vi "Fancy Swerve.vi"   [LabVIEW 2020]
uses:
  Robot Global Data.vi
  <vilib>/addons/control/pid/pid.llb/PID (DBL).vi
  <vilib>/addons/control/pid/NI_PID_pid.lvlib
types:
  T1 = cluster{"proportional gain (Kc)":dbl, "integral time (Ti, min)":dbl, "derivative time (Td, min)":dbl}
  T2 = typedef "WPI_MotorControlDeviceRef.ctl" = cluster{"DeviceStatus":errorcluster, "Type":T3, "PWM":cluster{"PWM Channel":T4, "DeadBand":T5}, "CAN":cluster{"Device Number":u8, "SetOutput VI Ref":variant, "GetOutput VI Ref":variant, "Enable VI Ref":variant, "Disable VI Ref":variant, "Data":variant}, "Invert":bool, "DIO PWM":cluster{"PWM \"Enable\" Channel":T4, "DIOChannel":T6, "PWM Rate":dbl}}
  T3 = typedef "WPI_MotorControlType.ctl" = enum16{"PWM", "CAN", "DIO PWM"}
  T4 = typedef "FPGA_DIOPWMChannel.ctl" = enum8{"PWM 0", "PWM 1", "PWM 2", "PWM 3", "PWM 4", "PWM 5", "PWM 6", "PWM 7", "PWM 8", "PWM 9", "PWM MXP 0", "PWM MXP 1", "PWM MXP 2", "PWM MXP 3", "PWM MXP 4", "PWM MXP 5", "PWM MXP 6", "PWM MXP 7", "PWM MXP 8", "PWM MXP 9", "Invalid"}
  T5 = typedef "WPI_PWMDeadband.ctl" = cluster{"Name":string, "maxPositivePwm":i32, "minPositivePwm":i32, "centerPwm":i32, "maxNegativePwm":i32, "minNegativePwm":i32, "angularRange":u16}
  T6 = typedef "FPGA_DIOChannel.ctl" = enum8{"DIO 0", "DIO 1", "DIO 2", "DIO 3", "DIO 4", "DIO 5", "DIO 6", "DIO 7", "DIO 8", "DIO 9", "DIO MXP 0", "DIO MXP 1", "DIO MXP 2", "DIO MXP 3", "DIO MXP 4", "DIO MXP 5", "DIO MXP 6", "DIO MXP 7", "DIO MXP 8", "DIO MXP 9", "DIO MXP 10", "DIO MXP 11", "DIO MXP 12", "DIO MXP 13", "DIO MXP 14", "DIO MXP 15", "SPI Port CS1", "SPI Port CS2", "SPI Port CS3", "SPI Port MISO", "SPI Port MOSI", "Invalid"}
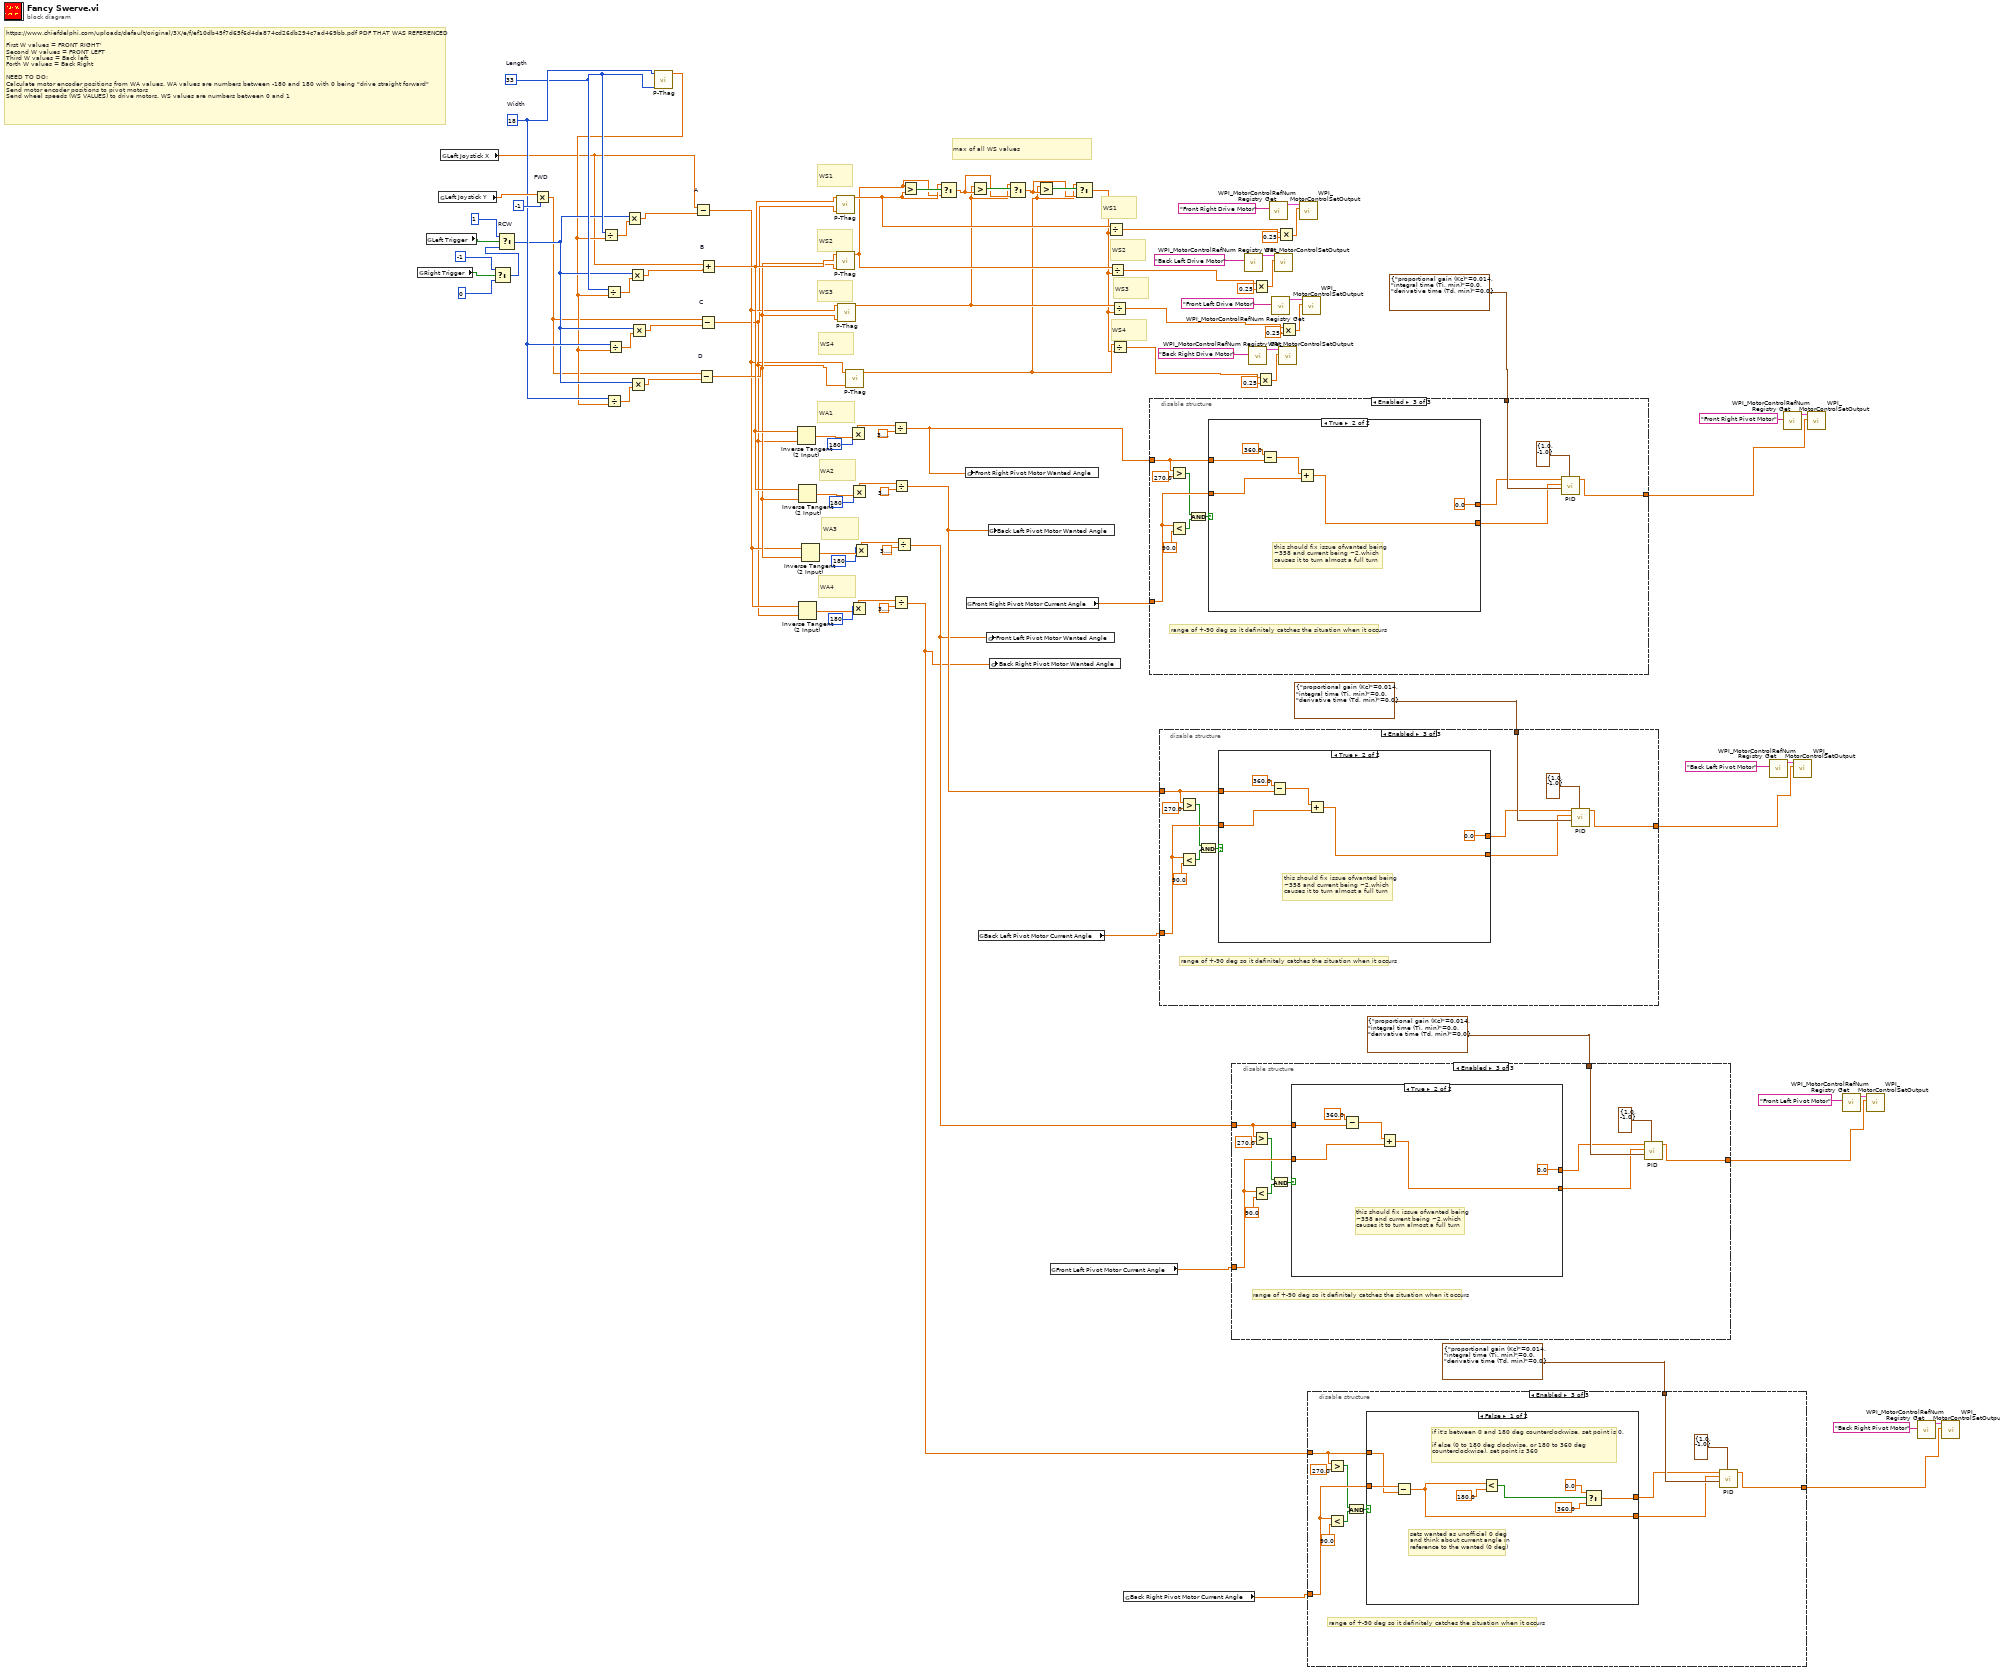
[diagram p0: block diagram]
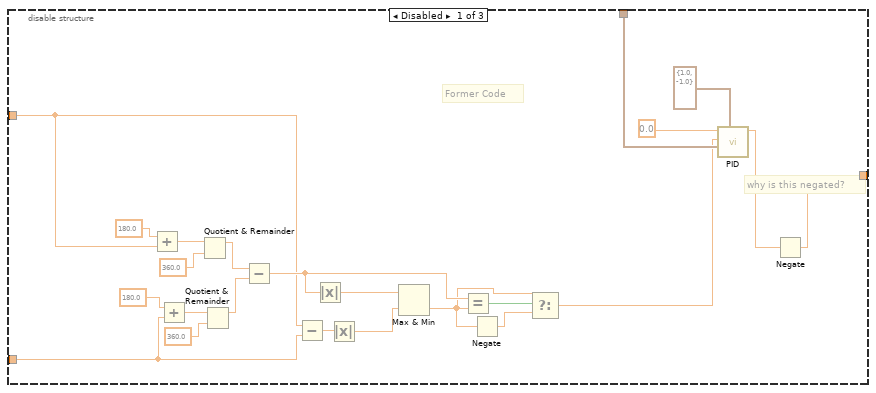
[diagram p2: hidden frame]
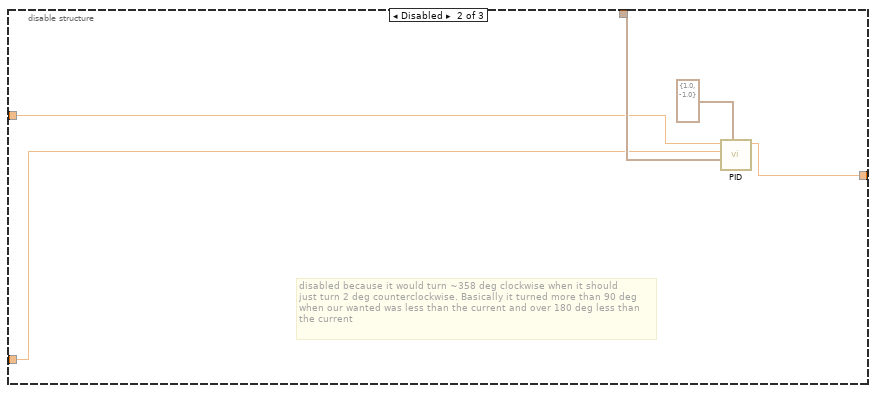
[diagram p3: hidden frame]
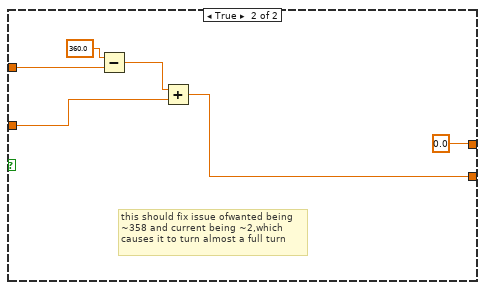
[diagram p4: hidden frame]
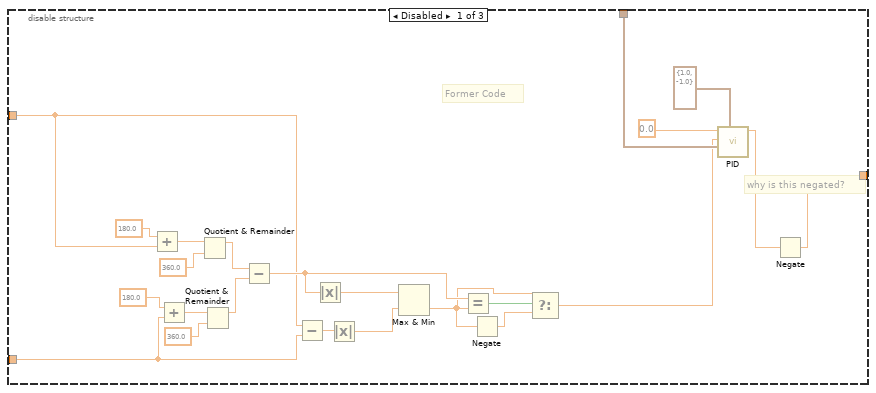
[diagram p5: hidden frame]
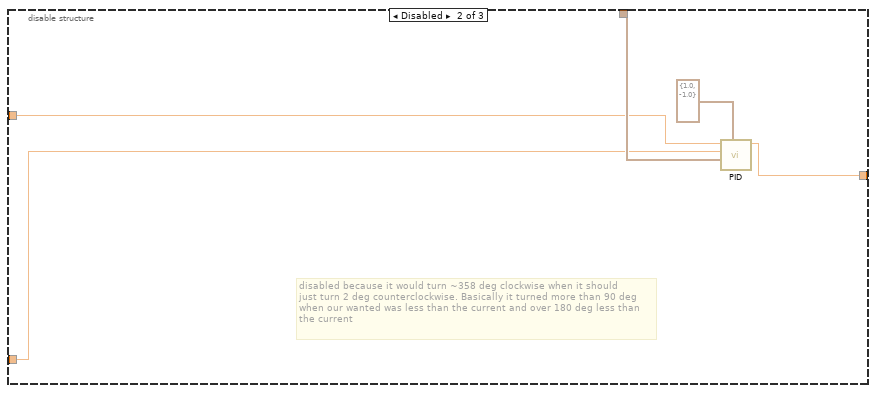
[diagram p6: hidden frame]
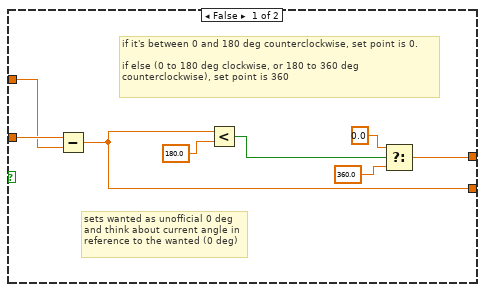
[diagram p7: hidden frame]
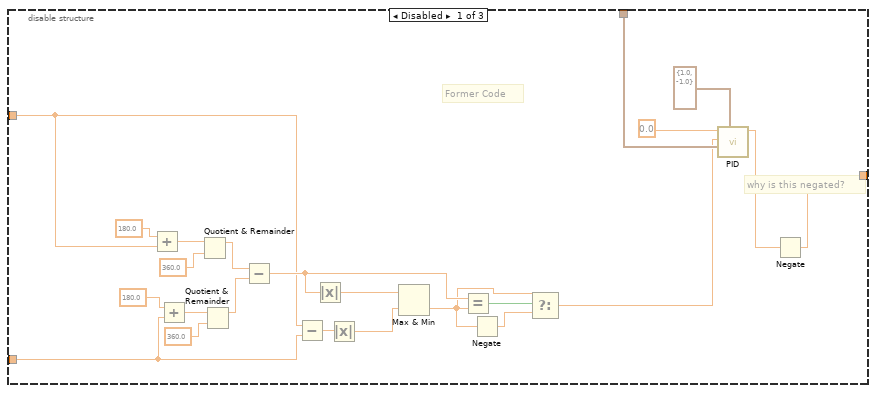
[diagram p8: hidden frame]
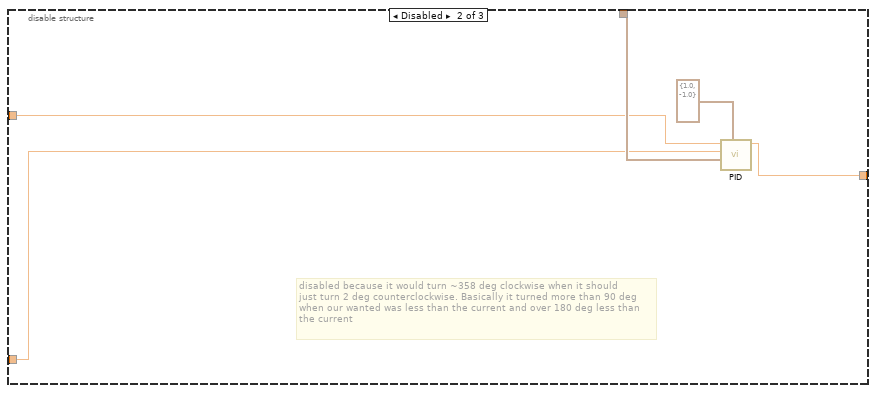
[diagram p9: hidden frame]
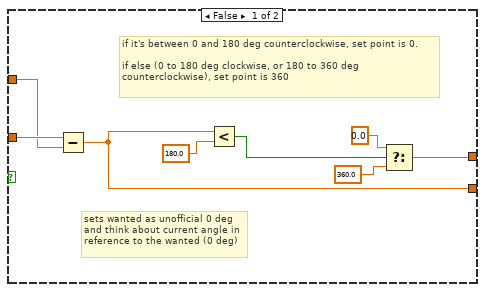
[diagram p10: hidden frame]
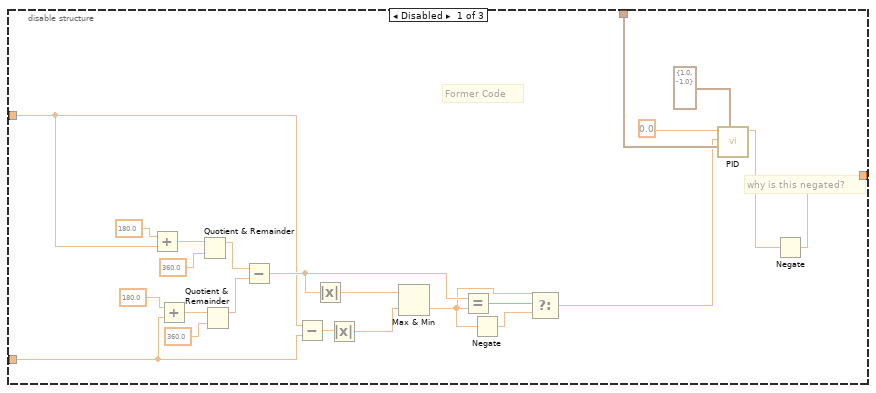
[diagram p11: hidden frame]
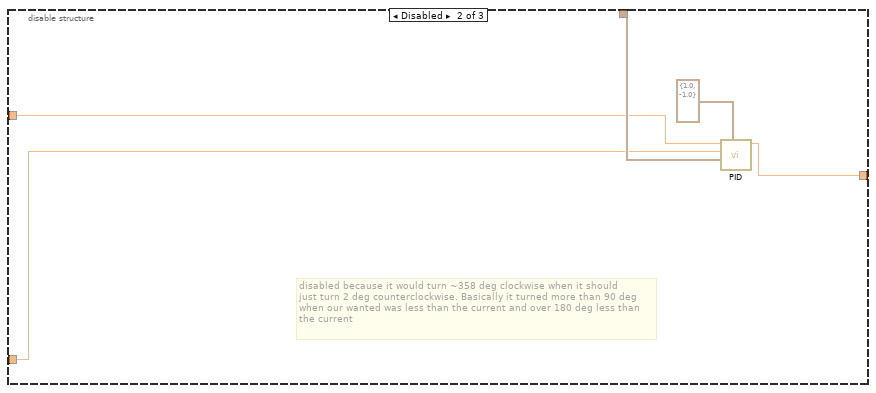
[diagram p12: hidden frame]
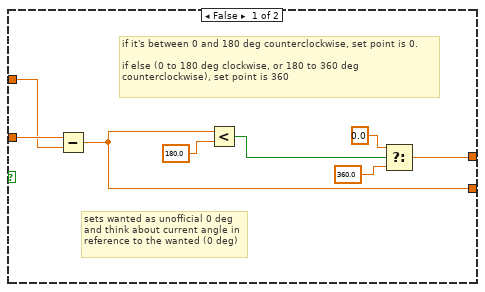
[diagram p13: hidden frame]
diagram:
  w79 = 33  # Length
  w80 = 18  # Width
  # "WS4"
  # "WS3"
  # "WS2"
  # "WS1"
  # "https://www.chiefdelphi.com/uploads/default/original/3X/e/f/ef10db45f7d65f6d4da874cd26db294c7ad469bb.pdf PDF THAT WAS REFERENCED\n\nFirst W values = FRONT RIGHT'\nSecond W values = FRONT LEFT\nThird W values = Back left\nForth W values = Back Right\n\nNEED TO DO:\nCalculate motor encoder positions from WA values. WA values are numbers between -180 and 180 with 0 being \"drive straight forward\"\nSend motor encoder positions to pivot motors\nSend wheel speeds (WS VALUES) to drive motors. WS values are numbers between 0 and 1"
  # "max of all WS values"
  # "WA4"
  # "WA3"
  # "WA2"
  # "WA1"
  # "WS4"
  # "WS3"
  # "WS2"
  # "WS1"
  n1 = global read "Robot Global Data.vi" "Right Trigger"() -> (w91:bool)
  n2 = global read "Robot Global Data.vi" "Left Trigger"() -> (w93:bool)
  n3 = global read "Robot Global Data.vi" "Left Joystick Y"() -> (w96:dbl)
  n4 = global read "Robot Global Data.vi" "Left Joystick X"() -> (w2:dbl)
  n5 = Select(t=-1, s=w91, f=0) -> (s? t:f=w92:i32)
  n6 = Select "RCW"(t=1, s=w93, f=w92) -> (s? t:f=w4:i32)
  n7 = Multiply "FWD"(x=w96, y=-1) -> (x*y=w1:dbl)
  n8 = call "P-Thag.vi"("Width"=w80, "Length"=w79) -> ("Output"=w3:dbl)  [unwired: 7 in]
  n9 = Divide(x=w79, y=w3) -> (x/y=w88:dbl)
  n10 = Divide(x=w79, y=w3) -> (x/y=w86:dbl)
  n11 = Divide(x=w80, y=w3) -> (x/y=w82:dbl)
  n12 = Divide(x=w80, y=w3) -> (x/y=w84:dbl)
  n13 = Multiply(x=w4, y=w88) -> (x*y=w87:dbl)
  n14 = Multiply(x=w4, y=w86) -> (x*y=w85:dbl)
  n15 = Multiply(x=w4, y=w82) -> (x*y=w81:dbl)
  n16 = Multiply(x=w4, y=w84) -> (x*y=w83:dbl)
  n17 = Subtract "A"(x=w2, y=w87) -> (x-y=w60:dbl)
  n18 = Subtract "D"(x=w1, y=w81) -> (x-y=w61:dbl)
  n19 = Subtract "C"(x=w1, y=w83) -> (x-y=w59:dbl)
  n20 = Add "B"(x=w2, y=w85) -> (x+y=w62:dbl)
  n21 = Inverse Tangent (2 Input)(1:w59, 2:w62) -> (0:w77:dbl)
  n22 = Inverse Tangent (2 Input)(1:w59, 2:w60) -> (0:w64:dbl)
  n23 = Inverse Tangent (2 Input)(1:w61, 2:w62) -> (0:w72:dbl)
  n24 = Inverse Tangent (2 Input)(1:w61, 2:w60) -> (0:w69:dbl)
  n25 = call "P-Thag.vi"("Width"=w62, "Length"=w59) -> ("Output"=w53:dbl)  [unwired: 7 in]
  n26 = call "P-Thag.vi"("Width"=w62, "Length"=w61) -> ("Output"=w52:dbl)  [unwired: 7 in]
  n27 = call "P-Thag.vi"("Width"=w60, "Length"=w61) -> ("Output"=w51:dbl)  [unwired: 7 in]
  n28 = call "P-Thag.vi"("Width"=w60, "Length"=w59) -> ("Output"=w50:dbl)  [unwired: 7 in]
  n29 = Multiply(x=180, y=w77) -> (x*y=w76:dbl)
  n30 = Multiply(x=180, y=w64) -> (x*y=w65:dbl)
  n31 = Multiply(x=180, y=w72) -> (x*y=w73:dbl)
  n32 = Multiply(x=180, y=w69) -> (x*y=w68:dbl)
  n33 = Divide(x=w76, y=3.141592653589793) -> (x/y=w28:dbl)
  n34 = Divide(x=w65, y=3.141592653589793) -> (x/y=w5:dbl)
  n35 = Divide(x=w73, y=3.141592653589793) -> (x/y=w7:dbl)
  n36 = Divide(x=w68, y=3.141592653589793) -> (x/y=w6:dbl)
  n37 = Greater?(x=w52, y=w53) -> (0:w58:bool)
  n38 = Select(t=w53, s=w58, f=w52) -> (s? t:f=w56:dbl)
  n39 = global write "Robot Global Data.vi" "Front Right Pivot Motor Wanted Angle"(w28) -> ()
  n40 = global read "Robot Global Data.vi" "Front Right Pivot Motor Current Angle"() -> (w48:dbl)
  n41 = Greater?(x=w51, y=w56) -> (0:w57:bool)
  n42 = global read "Robot Global Data.vi" "Back Left Pivot Motor Current Angle"() -> (w42:dbl)
  n43 = global write "Robot Global Data.vi" "Front Left Pivot Motor Wanted Angle"(w6) -> ()
  n44 = global write "Robot Global Data.vi" "Back Left Pivot Motor Wanted Angle"(w7) -> ()
  n45 = global write "Robot Global Data.vi" "Back Right Pivot Motor Wanted Angle"(w5) -> ()
  n46 = Select(t=w51, s=w57, f=w56) -> (s? t:f=w54:dbl)
  n47 = Greater?(x=w50, y=w54) -> (0:w55:bool)
  n48 = global read "Robot Global Data.vi" "Front Left Pivot Motor Current Angle"() -> (w37:dbl)
  n49 = Select(t=w50, s=w55, f=w54) -> (s? t:f=w49:dbl)
  n50 = Divide(x=w53, y=w49) -> (x/y=w23:dbl)
  n51 = Divide(x=w52, y=w49) -> (x/y=w18:dbl)
  n52 = Divide(x=w51, y=w49) -> (x/y=w13:dbl)
  n53 = Divide(x=w50, y=w49) -> (x/y=w8:dbl)
  n54 = global read "Robot Global Data.vi" "Back Right Pivot Motor Current Angle"() -> (w32:dbl)
  n55 = disable-structure shown="Enabled" {
    disable-tunnel: T1 {"proportional gain (Kc)"=0.014, "integral time (Ti, min)"=0.0, "derivative time (Td, min)"=0.0} ("FR Pivot Motor PID gains") -> [w119 w123 w135]
    disable-tunnel: w48 -> [w116 w121 w129]
    disable-tunnel: w28 -> [w98 w122 w131]
    disable-tunnel: [w97 w120 w134] -> w44
    frame Disabled {
      # "why is this negated?"
      # "Former Code"
      n56 = Add(x=180.0, y=w98) -> (x+y=w110:dbl)
      n57 = Add(x=180.0, y=w116) -> (x+y=w108:dbl)
      n58 = Quotient & Remainder(x=w110, y=360.0) -> (x-y*floor(x/y)=w106:dbl)  [unwired: 1 out]
      n59 = Quotient & Remainder(x=w108, y=360.0) -> (x-y*floor(x/y)=w105:dbl)  [unwired: 1 out]
      n60 = Subtract(x=w106, y=w105) -> (x-y=w104:dbl)
      n61 = Subtract(x=w98, y=w116) -> (x-y=w103:dbl)
      n62 = Absolute Value(x=w104) -> (abs(x)=w102:dbl)
      n63 = Absolute Value(x=w103) -> (abs(x)=w101:dbl)
      n64 = Max & Min(x=w102, y=w101) -> (min(x,y)=w100:dbl)  [unwired: 1 out]
      n65 = Equal?(x=w104, y=w100) -> (x = y?=w111:bool)
      n66 = Negate(x=w100) -> (-x=w112:dbl)
      n67 = Select(t=w100, s=w111, f=w112) -> (s? t:f=w113:dbl)
      n68 = call-poly <vilib>:"PID.vi"("output range"=cluster{"output high":dbl, "output low":dbl} {"output high"=1.0, "output low"=-1.0}, "PID gains"=w119, "process variable"=w113, "setpoint"=0.0) -> ("output"=w99:dbl)  [unwired: 6 in, 1 out]
      n69 = Negate(x=w99) -> (-x=w97:dbl)
    }
    frame Disabled {
      # "disabled because it would turn ~358 deg clockwise when it should \njust turn 2 deg counterclockwise. Basically it turned more than 90 deg\nwhen our wanted was less than the current and over 180 deg less than\nthe current"
      n70 = call-poly <vilib>:"PID.vi"("output range"=cluster{"output high":dbl, "output low":dbl} {"output high"=1.0, "output low"=-1.0}, "PID gains"=w123, "process variable"=w121, "setpoint"=w122) -> ("output"=w120:dbl)  [unwired: 6 in, 1 out]
    }
    frame Enabled {
      # "range of +-90 deg so it definitely catches the situation when it occurs"
      n71 = Greater?(x=w131, y=270.0) -> (0:w125:bool)
      n72 = Less?(x=w129, y=90.0) -> (x < y?=w126:bool)
      n73 = And(x=w125, y=w126) -> (x .and. y?=w127:bool)
      n74 = case shown="True" w127 {
        tunnel: [w144 0.0] -> w133
        tunnel: w129 -> [w139 w147]
        tunnel: w131 -> [w138 w150]
        tunnel: [w137 w146] -> w132
        frame False {
          # "if it's between 0 and 180 deg counterclockwise, set point is 0.\n \nif else (0 to 180 deg clockwise, or 180 to 360 deg \ncounterclockwise), set point is 360"
          # "sets wanted as unofficial 0 deg\nand think about current angle in\nreference to the wanted (0 deg)"
          n75 = Subtract(x=w139, y=w138) -> (x-y=w137:dbl)
          n76 = Less?(x=w137, y=180.0 ("upper limit")) -> (x < y?=w143:bool)
          n77 = Select(t=0.0, s=w143, f=360.0) -> (s? t:f=w144:dbl)
        }
        frame True {
          # "this should fix issue ofwanted being\n~358 and current being ~2,which \ncauses it to turn almost a full turn"
          n78 = Subtract(x=360.0, y=w150) -> (x-y=w148:dbl)
          n79 = Add(x=w148, y=w147) -> (x+y=w146:dbl)
        }
      }
      n80 = call-poly <vilib>:"PID.vi"("output range"=cluster{"output high":dbl, "output low":dbl} {"output high"=1.0, "output low"=-1.0}, "PID gains"=w135, "process variable"=w132, "setpoint"=w133) -> ("output"=w134:dbl)  [unwired: 6 in, 1 out]
    }
  }
  n81 = disable-structure shown="Enabled" {
    disable-tunnel: T1 {"proportional gain (Kc)"=0.014, "integral time (Ti, min)"=0.0, "derivative time (Td, min)"=0.0} ("FR Pivot Motor PID gains") -> [w173 w177 w189]
    disable-tunnel: w42 -> [w170 w175 w183]
    disable-tunnel: w7 -> [w152 w176 w185]
    disable-tunnel: [w151 w174 w188] -> w39
    frame Disabled {
      # "why is this negated?"
      # "Former Code"
      n82 = Add(x=180.0, y=w152) -> (x+y=w164:dbl)
      n83 = Add(x=180.0, y=w170) -> (x+y=w162:dbl)
      n84 = Quotient & Remainder(x=w164, y=360.0) -> (x-y*floor(x/y)=w160:dbl)  [unwired: 1 out]
      n85 = Quotient & Remainder(x=w162, y=360.0) -> (x-y*floor(x/y)=w159:dbl)  [unwired: 1 out]
      n86 = Subtract(x=w160, y=w159) -> (x-y=w158:dbl)
      n87 = Subtract(x=w152, y=w170) -> (x-y=w157:dbl)
      n88 = Absolute Value(x=w158) -> (abs(x)=w156:dbl)
      n89 = Absolute Value(x=w157) -> (abs(x)=w155:dbl)
      n90 = Max & Min(x=w156, y=w155) -> (min(x,y)=w154:dbl)  [unwired: 1 out]
      n91 = Equal?(x=w158, y=w154) -> (x = y?=w165:bool)
      n92 = Negate(x=w154) -> (-x=w166:dbl)
      n93 = Select(t=w154, s=w165, f=w166) -> (s? t:f=w167:dbl)
      n94 = call-poly <vilib>:"PID.vi"("output range"=cluster{"output high":dbl, "output low":dbl} {"output high"=1.0, "output low"=-1.0}, "PID gains"=w173, "process variable"=w167, "setpoint"=0.0) -> ("output"=w153:dbl)  [unwired: 6 in, 1 out]
      n95 = Negate(x=w153) -> (-x=w151:dbl)
    }
    frame Disabled {
      # "disabled because it would turn ~358 deg clockwise when it should \njust turn 2 deg counterclockwise. Basically it turned more than 90 deg\nwhen our wanted was less than the current and over 180 deg less than\nthe current"
      n96 = call-poly <vilib>:"PID.vi"("output range"=cluster{"output high":dbl, "output low":dbl} {"output high"=1.0, "output low"=-1.0}, "PID gains"=w177, "process variable"=w175, "setpoint"=w176) -> ("output"=w174:dbl)  [unwired: 6 in, 1 out]
    }
    frame Enabled {
      # "range of +-90 deg so it definitely catches the situation when it occurs"
      n97 = Greater?(x=w185, y=270.0) -> (0:w179:bool)
      n98 = Less?(x=w183, y=90.0) -> (x < y?=w180:bool)
      n99 = And(x=w179, y=w180) -> (x .and. y?=w181:bool)
      n100 = case shown="True" w181 {
        tunnel: [w198 0.0] -> w187
        tunnel: w183 -> [w193 w201]
        tunnel: w185 -> [w192 w204]
        tunnel: [w191 w200] -> w186
        frame False {
          # "if it's between 0 and 180 deg counterclockwise, set point is 0.\n \nif else (0 to 180 deg clockwise, or 180 to 360 deg \ncounterclockwise), set point is 360"
          # "sets wanted as unofficial 0 deg\nand think about current angle in\nreference to the wanted (0 deg)"
          n101 = Subtract(x=w193, y=w192) -> (x-y=w191:dbl)
          n102 = Less?(x=w191, y=180.0 ("upper limit")) -> (x < y?=w197:bool)
          n103 = Select(t=0.0, s=w197, f=360.0) -> (s? t:f=w198:dbl)
        }
        frame True {
          # "this should fix issue ofwanted being\n~358 and current being ~2,which \ncauses it to turn almost a full turn"
          n104 = Subtract(x=360.0, y=w204) -> (x-y=w202:dbl)
          n105 = Add(x=w202, y=w201) -> (x+y=w200:dbl)
        }
      }
      n106 = call-poly <vilib>:"PID.vi"("output range"=cluster{"output high":dbl, "output low":dbl} {"output high"=1.0, "output low"=-1.0}, "PID gains"=w189, "process variable"=w186, "setpoint"=w187) -> ("output"=w188:dbl)  [unwired: 6 in, 1 out]
    }
  }
  n107 = disable-structure shown="Enabled" {
    disable-tunnel: T1 {"proportional gain (Kc)"=0.014, "integral time (Ti, min)"=0.0, "derivative time (Td, min)"=0.0} ("FR Pivot Motor PID gains") -> [w227 w231 w243]
    disable-tunnel: w37 -> [w224 w229 w237]
    disable-tunnel: w6 -> [w206 w230 w239]
    disable-tunnel: [w205 w228 w242] -> w34
    frame Disabled {
      # "why is this negated?"
      # "Former Code"
      n108 = Add(x=180.0, y=w206) -> (x+y=w218:dbl)
      n109 = Add(x=180.0, y=w224) -> (x+y=w216:dbl)
      n110 = Quotient & Remainder(x=w218, y=360.0) -> (x-y*floor(x/y)=w214:dbl)  [unwired: 1 out]
      n111 = Quotient & Remainder(x=w216, y=360.0) -> (x-y*floor(x/y)=w213:dbl)  [unwired: 1 out]
      n112 = Subtract(x=w214, y=w213) -> (x-y=w212:dbl)
      n113 = Subtract(x=w206, y=w224) -> (x-y=w211:dbl)
      n114 = Absolute Value(x=w212) -> (abs(x)=w210:dbl)
      n115 = Absolute Value(x=w211) -> (abs(x)=w209:dbl)
      n116 = Max & Min(x=w210, y=w209) -> (min(x,y)=w208:dbl)  [unwired: 1 out]
      n117 = Equal?(x=w212, y=w208) -> (x = y?=w219:bool)
      n118 = Negate(x=w208) -> (-x=w220:dbl)
      n119 = Select(t=w208, s=w219, f=w220) -> (s? t:f=w221:dbl)
      n120 = call-poly <vilib>:"PID.vi"("output range"=cluster{"output high":dbl, "output low":dbl} {"output high"=1.0, "output low"=-1.0}, "PID gains"=w227, "process variable"=w221, "setpoint"=0.0) -> ("output"=w207:dbl)  [unwired: 6 in, 1 out]
      n121 = Negate(x=w207) -> (-x=w205:dbl)
    }
    frame Disabled {
      # "disabled because it would turn ~358 deg clockwise when it should \njust turn 2 deg counterclockwise. Basically it turned more than 90 deg\nwhen our wanted was less than the current and over 180 deg less than\nthe current"
      n122 = call-poly <vilib>:"PID.vi"("output range"=cluster{"output high":dbl, "output low":dbl} {"output high"=1.0, "output low"=-1.0}, "PID gains"=w231, "process variable"=w229, "setpoint"=w230) -> ("output"=w228:dbl)  [unwired: 6 in, 1 out]
    }
    frame Enabled {
      # "range of +-90 deg so it definitely catches the situation when it occurs"
      n123 = Greater?(x=w239, y=270.0) -> (0:w233:bool)
      n124 = Less?(x=w237, y=90.0) -> (x < y?=w234:bool)
      n125 = And(x=w233, y=w234) -> (x .and. y?=w235:bool)
      n126 = case shown="True" w235 {
        tunnel: [w252 0.0] -> w241
        tunnel: w237 -> [w247 w255]
        tunnel: w239 -> [w246 w258]
        tunnel: [w245 w254] -> w240
        frame False {
          # "if it's between 0 and 180 deg counterclockwise, set point is 0.\n \nif else (0 to 180 deg clockwise, or 180 to 360 deg \ncounterclockwise), set point is 360"
          # "sets wanted as unofficial 0 deg\nand think about current angle in\nreference to the wanted (0 deg)"
          n127 = Subtract(x=w247, y=w246) -> (x-y=w245:dbl)
          n128 = Less?(x=w245, y=180.0 ("upper limit")) -> (x < y?=w251:bool)
          n129 = Select(t=0.0, s=w251, f=360.0) -> (s? t:f=w252:dbl)
        }
        frame True {
          # "this should fix issue ofwanted being\n~358 and current being ~2,which \ncauses it to turn almost a full turn"
          n130 = Subtract(x=360.0, y=w258) -> (x-y=w256:dbl)
          n131 = Add(x=w256, y=w255) -> (x+y=w254:dbl)
        }
      }
      n132 = call-poly <vilib>:"PID.vi"("output range"=cluster{"output high":dbl, "output low":dbl} {"output high"=1.0, "output low"=-1.0}, "PID gains"=w243, "process variable"=w240, "setpoint"=w241) -> ("output"=w242:dbl)  [unwired: 6 in, 1 out]
    }
  }
  n133 = call <vilib>:"WPI_MotorControlRefNum Registry Get.vi"("refnum name"="Back Left Drive Motor") -> ("MotorControlDevRef"=w22:T2)  [unwired: 9 in, 1 out]
  n134 = call <vilib>:"WPI_MotorControlRefNum Registry Get.vi"("refnum name"="Back Right Drive Motor") -> ("MotorControlDevRef"=w12:T2)  [unwired: 9 in, 1 out]
  n135 = Multiply(x=w18, y=0.25) -> (x*y=w20:dbl)
  n136 = Multiply(x=w8, y=0.25) -> (x*y=w10:dbl)
  n137 = call <vilib>:"WPI_MotorControlRefNum Registry Get.vi"("refnum name"="Front Right Drive Motor") -> ("MotorControlDevRef"=w27:T2)  [unwired: 9 in, 1 out]
  n138 = call <vilib>:"WPI_MotorControlRefNum Registry Get.vi"("refnum name"="Front Left Drive Motor") -> ("MotorControlDevRef"=w17:T2)  [unwired: 9 in, 1 out]
  n139 = call <vilib>:"WPI_MotorControlSetOutput.vi"("Output"=w20, "MotorControlDevRef"=w22) -> ()  [unwired: 7 in, 3 out]
  n140 = Multiply(x=w23, y=0.25) -> (x*y=w25:dbl)
  n141 = call <vilib>:"WPI_MotorControlSetOutput.vi"("Output"=w10, "MotorControlDevRef"=w12) -> ()  [unwired: 7 in, 3 out]
  n142 = Multiply(x=w13, y=0.25) -> (x*y=w15:dbl)
  n143 = call <vilib>:"WPI_MotorControlSetOutput.vi"("Output"=w25, "MotorControlDevRef"=w27) -> ()  [unwired: 7 in, 3 out]
  n144 = call <vilib>:"WPI_MotorControlSetOutput.vi"("Output"=w15, "MotorControlDevRef"=w17) -> ()  [unwired: 7 in, 3 out]
  n145 = disable-structure shown="Enabled" {
    disable-tunnel: T1 {"proportional gain (Kc)"=0.014, "integral time (Ti, min)"=0.0, "derivative time (Td, min)"=0.0} ("FR Pivot Motor PID gains") -> [w281 w285 w297]
    disable-tunnel: w32 -> [w278 w283 w291]
    disable-tunnel: w5 -> [w260 w284 w293]
    disable-tunnel: [w259 w282 w296] -> w29
    frame Disabled {
      # "why is this negated?"
      # "Former Code"
      n146 = Add(x=180.0, y=w260) -> (x+y=w272:dbl)
      n147 = Add(x=180.0, y=w278) -> (x+y=w270:dbl)
      n148 = Quotient & Remainder(x=w272, y=360.0) -> (x-y*floor(x/y)=w268:dbl)  [unwired: 1 out]
      n149 = Quotient & Remainder(x=w270, y=360.0) -> (x-y*floor(x/y)=w267:dbl)  [unwired: 1 out]
      n150 = Subtract(x=w268, y=w267) -> (x-y=w266:dbl)
      n151 = Subtract(x=w260, y=w278) -> (x-y=w265:dbl)
      n152 = Absolute Value(x=w266) -> (abs(x)=w264:dbl)
      n153 = Absolute Value(x=w265) -> (abs(x)=w263:dbl)
      n154 = Max & Min(x=w264, y=w263) -> (min(x,y)=w262:dbl)  [unwired: 1 out]
      n155 = Equal?(x=w266, y=w262) -> (x = y?=w273:bool)
      n156 = Negate(x=w262) -> (-x=w274:dbl)
      n157 = Select(t=w262, s=w273, f=w274) -> (s? t:f=w275:dbl)
      n158 = call-poly <vilib>:"PID.vi"("output range"=cluster{"output high":dbl, "output low":dbl} {"output high"=1.0, "output low"=-1.0}, "PID gains"=w281, "process variable"=w275, "setpoint"=0.0) -> ("output"=w261:dbl)  [unwired: 6 in, 1 out]
      n159 = Negate(x=w261) -> (-x=w259:dbl)
    }
    frame Disabled {
      # "disabled because it would turn ~358 deg clockwise when it should \njust turn 2 deg counterclockwise. Basically it turned more than 90 deg\nwhen our wanted was less than the current and over 180 deg less than\nthe current"
      n160 = call-poly <vilib>:"PID.vi"("output range"=cluster{"output high":dbl, "output low":dbl} {"output high"=1.0, "output low"=-1.0}, "PID gains"=w285, "process variable"=w283, "setpoint"=w284) -> ("output"=w282:dbl)  [unwired: 6 in, 1 out]
    }
    frame Enabled {
      # "range of +-90 deg so it definitely catches the situation when it occurs"
      n161 = Greater?(x=w293, y=270.0) -> (0:w287:bool)
      n162 = Less?(x=w291, y=90.0) -> (x < y?=w288:bool)
      n163 = And(x=w287, y=w288) -> (x .and. y?=w289:bool)
      n164 = case shown="False" w289 {
        tunnel: [w306 0.0] -> w295
        tunnel: w291 -> [w301 w309]
        tunnel: w293 -> [w300 w312]
        tunnel: [w299 w308] -> w294
        frame False {
          # "if it's between 0 and 180 deg counterclockwise, set point is 0.\n \nif else (0 to 180 deg clockwise, or 180 to 360 deg \ncounterclockwise), set point is 360"
          # "sets wanted as unofficial 0 deg\nand think about current angle in\nreference to the wanted (0 deg)"
          n165 = Subtract(x=w301, y=w300) -> (x-y=w299:dbl)
          n166 = Less?(x=w299, y=180.0 ("upper limit")) -> (x < y?=w305:bool)
          n167 = Select(t=0.0, s=w305, f=360.0) -> (s? t:f=w306:dbl)
        }
        frame True {
          # "this should fix issue ofwanted being\n~358 and current being ~2,which \ncauses it to turn almost a full turn"
          n168 = Subtract(x=360.0, y=w312) -> (x-y=w310:dbl)
          n169 = Add(x=w310, y=w309) -> (x+y=w308:dbl)
        }
      }
      n170 = call-poly <vilib>:"PID.vi"("output range"=cluster{"output high":dbl, "output low":dbl} {"output high"=1.0, "output low"=-1.0}, "PID gains"=w297, "process variable"=w294, "setpoint"=w295) -> ("output"=w296:dbl)  [unwired: 6 in, 1 out]
    }
  }
  n171 = call <vilib>:"WPI_MotorControlRefNum Registry Get.vi"("refnum name"="Back Left Pivot Motor") -> ("MotorControlDevRef"=w40:T2)  [unwired: 9 in, 1 out]
  n172 = call <vilib>:"WPI_MotorControlRefNum Registry Get.vi"("refnum name"="Front Right Pivot Motor") -> ("MotorControlDevRef"=w45:T2)  [unwired: 9 in, 1 out]
  n173 = call <vilib>:"WPI_MotorControlSetOutput.vi"("Output"=w39, "MotorControlDevRef"=w40) -> ()  [unwired: 7 in, 3 out]
  n174 = call <vilib>:"WPI_MotorControlSetOutput.vi"("Output"=w44, "MotorControlDevRef"=w45) -> ()  [unwired: 7 in, 3 out]
  n175 = call <vilib>:"WPI_MotorControlRefNum Registry Get.vi"("refnum name"="Front Left Pivot Motor") -> ("MotorControlDevRef"=w35:T2)  [unwired: 9 in, 1 out]
  n176 = call <vilib>:"WPI_MotorControlSetOutput.vi"("Output"=w34, "MotorControlDevRef"=w35) -> ()  [unwired: 7 in, 3 out]
  n177 = call <vilib>:"WPI_MotorControlRefNum Registry Get.vi"("refnum name"="Back Right Pivot Motor") -> ("MotorControlDevRef"=w30:T2)  [unwired: 9 in, 1 out]
  n178 = call <vilib>:"WPI_MotorControlSetOutput.vi"("Output"=w29, "MotorControlDevRef"=w30) -> ()  [unwired: 7 in, 3 out]
